vi "LEDStateControl.vi"   [LabVIEW 2018]
uses:
  RefNumsDriverStation.vi
  Robot States.vi
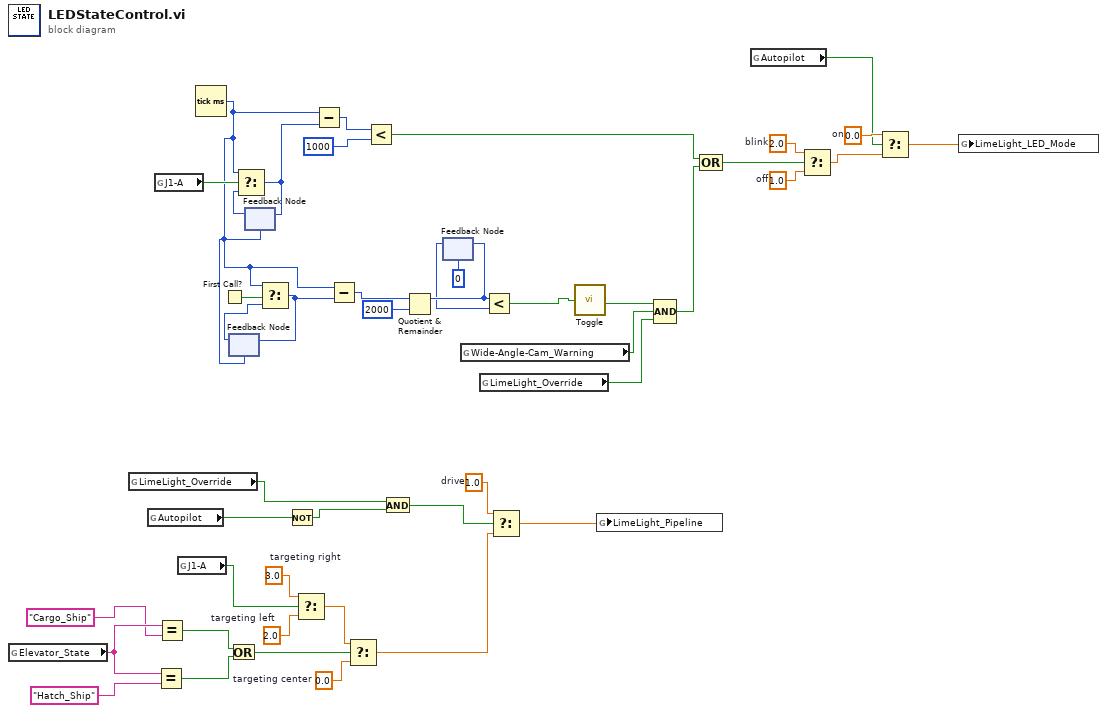
[diagram p0: block diagram]
diagram:
  w5 = 1.0  # drive
  w11 = 0.0  # targeting center
  w13 = 2.0  # targeting left
  w14 = 3.0  # targeting right
  w24 = 0.0  # on
  w26 = 1.0  # off
  w27 = 2.0  # blink
  n1 = global read "Robot States.vi" "Elevator_State"() -> (w21:string)
  n2 = global read "RefNumsDriverStation.vi" "LimeLight_Override"() -> (w7:bool)
  n3 = global read "Robot States.vi" "Autopilot"() -> (w9:bool)
  n4 = global read "RefNumsDriverStation.vi" "J1-A"() -> (w42:bool)
  n5 = Equal?(x=w21, y="Hatch_Ship") -> (x = y?=w17:bool)
  n6 = Equal?(x=w21, y="Cargo_Ship") -> (x = y?=w18:bool)
  n7 = global read "RefNumsDriverStation.vi" "J1-A"() -> (w15:bool)
  n8 = Tick Count (ms)() -> (millisecond timer value=w3:u32)
  n9 = First Call?() -> (First Call?: T/F=w41:bool)
  n10 = feedback #1(w3) -> (w40:u32)
  n11 = Or(x=w18, y=w17) -> (x .or. y?=w16:bool)
  n12 = feedback #2(w3) -> (w39:u32)
  n13 = Select(t=w3, s=w42, f=w39) -> (s? t:f=w43:u32)
  n14 = feedback-in #2(w43) -> ()
  n15 = Select(t=w3, s=w41, f=w40) -> (s? t:f=w38:u32)
  n16 = feedback-in #1(w38) -> ()
  n17 = Not(x=w9) -> (.not. x?=w8:bool)
  n18 = Select(t=w14, s=w15, f=w13) -> (s? t:f=w12:dbl)
  n19 = Subtract(x=w3, y=w43) -> (x-y=w45:u32)
  n20 = Subtract(x=w3, y=w38) -> (x-y=w37:u32)
  n21 = Select(t=w12, s=w16, f=w11) -> (s? t:f=w10:dbl)
  n22 = Less?(x=w45, y=u32 1000) -> (x < y?=w29:bool)
  n23 = And(x=w7, y=w8) -> (x .and. y?=w6:bool)
  n24 = Quotient & Remainder(x=w37, y=u32 2000) -> (x-y*floor(x/y)=w35:u32)  [unwired: 1 out]
  n25 = feedback #3(u32 0) -> (w34:u32)
  n26 = feedback-in #3(w35) -> ()
  n27 = global read "RefNumsDriverStation.vi" "Wide-Angle-Cam_Warning"() -> (w32:bool)
  n28 = global read "RefNumsDriverStation.vi" "LimeLight_Override"() -> (w31:bool)
  n29 = Less?(x=w35, y=w34) -> (x < y?=w2:bool)
  n30 = Select(t=w5, s=w6, f=w10) -> (s? t:f=w4:dbl)
  n31 = call "Toggle.vi"("Trigger"=w2) -> ("New_Mode"=w1:bool)
  n32 = global write "Robot States.vi" "LimeLight_Pipeline"(w4) -> ()
  n33 = Compound Arithmetic op=AND(w1, w32, w31) -> (w30:bool)
  n34 = Compound Arithmetic op=OR(w29, w30) -> (w28:bool)
  n35 = global read "Robot States.vi" "Autopilot"() -> (w23:bool)
  n36 = Select(t=w27, s=w28, f=w26) -> (s? t:f=w25:dbl)
  n37 = Select(t=w24, s=w23, f=w25) -> (s? t:f=w22:dbl)
  n38 = global write "Robot States.vi" "LimeLight_LED_Mode"(w22) -> ()
